vi "Load.vi"(8 "error in (no error)":errorcluster, 11 "User Preferences File in":refnum<class "User Preferences File.lvclass">) -> (0 "error out":errorcluster, 3 "User Preferences File out":refnum<class "User Preferences File.lvclass">)   [LabVIEW 2020, in "User Preferences File.lvclass"]
doc: "Load the preferences file from disk into memory. The loaded file can be accessed through the appropriate accessor members. The initialization member VI should be executed before this VI is run."
uses:
  User Preferences File.lvclass
  User Preferences Cluster.ctl
  User Preferences File.lvclass/User Preferences File.ctl
panel:
  out "User Preferences":T1={"Max Recent Experiments"=30.0, "Recent Experiments"=[]}
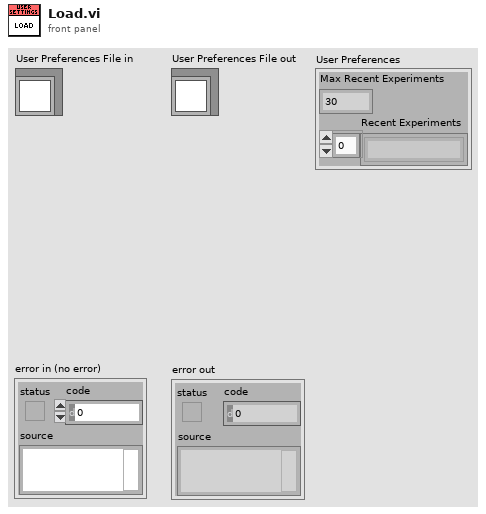
[diagram p1: front panel]
types:
  T1 = typedef "User Preferences File.lvclass/User Preferences Cluster.ctl" = cluster{"Max Recent Experiments":dbl, "Recent Experiments":string[]}
  T2 = enum16{"open", "replace", "create", "open or create", "replace or create", "replace or create with confirmation"}
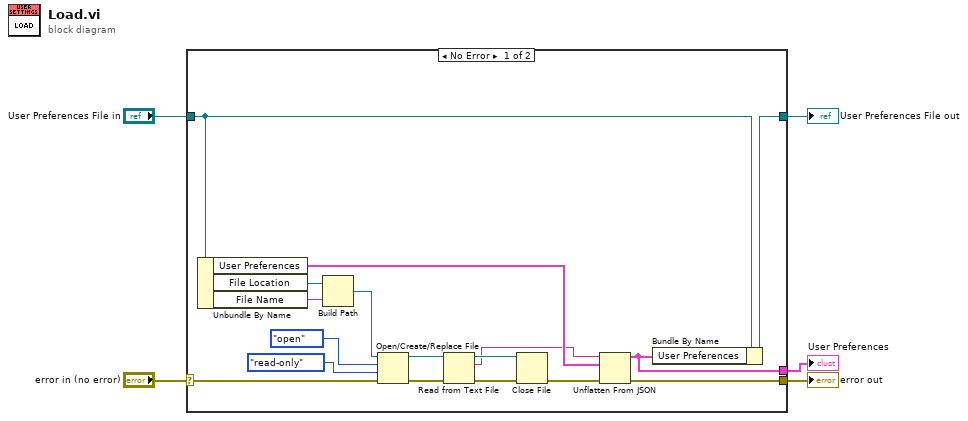
[diagram p0: block diagram]
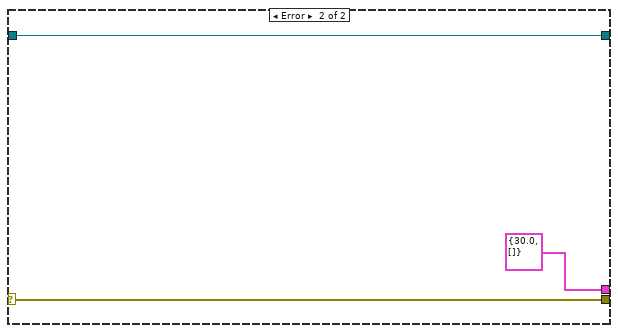
[diagram p2: hidden frame]
diagram:
  n1 = case shown="No Error" "error in (no error)" {
    selector: "error in (no error)" -> [w22 w25]
    tunnel: [w15 w25] -> w4
    tunnel: [w8 w24] -> w2
    tunnel: "User Preferences File in" -> [w14 w24]
    tunnel: [w7 T1 {"Max Recent Experiments"=30.0, "Recent Experiments"=[]} ("User Preferences")] -> w1
    frame No Error {
      n2 = Unbundle By Name(w14) -> ("User Preferences"=w13:T1, "File Location"=w11:path, "File Name"=w10:string)
      n3 = Build Path(base path=w11, name or relative path=w10) -> (appended path=w9:path)
      n4 = Open/Create/Replace File(file path (use dialog)=w9, error in=w22, operation (0:open)=T2."open", access (0:read/write)=enum16{"read/write", "read-only", "write-only"}."read-only") -> (refnum out=w19:refnum<file>, error out=w21:errorcluster)  [unwired: 2 in, 1 out]
      n5 = Read from Text File(file (use dialog)=w19, error in=w21) -> (refnum out=w17:refnum<file>, text=w12:string, error out=w20:errorcluster)  [unwired: 2 in, 1 out]
      n6 = Close File(refnum=w17, error in=w20) -> (error out=w16:errorcluster)  [unwired: 1 out]
      n7 = Unflatten From JSON(JSON string=w12, type and defaults=w13, error in (no error)=w16) -> (value=w7:T1, error out=w15:errorcluster)  [unwired: 4 in]
      n8 = Bundle By Name(cluster=w14, "User Preferences"=w7) -> (w8:refnum<class "User Preferences File.lvclass">)
    }
    frame Error {
    }
  }
  "error out" <- w4
  "User Preferences File out" <- w2
  "User Preferences" <- w1
